vi "Echo.vi"(8 "error in (no error)":errorcluster, 10 "Error In":errorcluster, 11 "HandlerCore in":refnum<class "HandlerCore.lvclass">) -> (0 "error out":errorcluster, 1 "Still Pass?":bool, 2 "handled?":bool, 3 "HandlerCore out":refnum<class "HandlerCore.lvclass">)   [LabVIEW 2014, in "Chain Of Responsibility Pattern.lvlib" / "HandlerCore.lvclass"]
uses:
  HandlerCore.lvclass
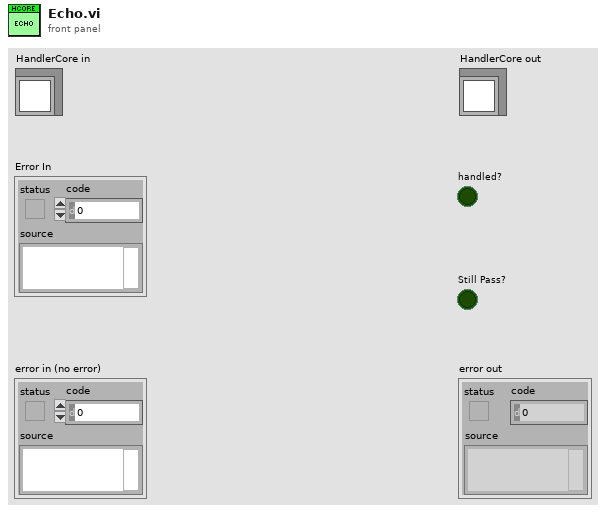
[diagram p1: front panel]
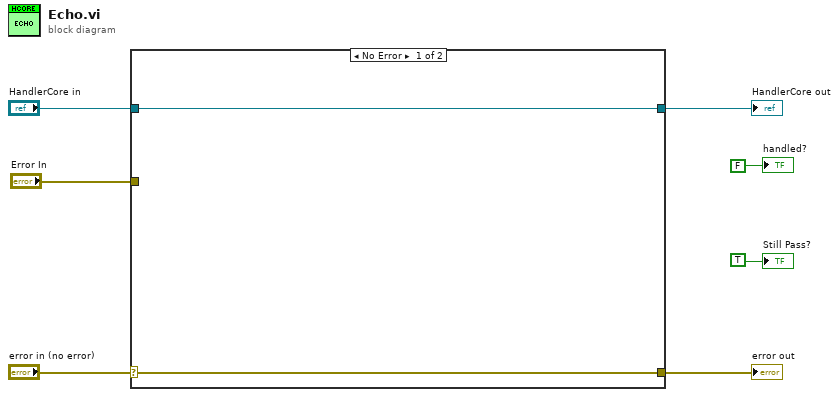
[diagram p0: block diagram]
diagram:
  n1 = case shown="No Error" "error in (no error)" {
    selector: "error in (no error)" -> [w8 w11]
    tunnel: [w8 w11] -> w6
    tunnel: [w9 w10] -> w4
    tunnel: "HandlerCore in" -> [w9 w10]
    tunnel: "Error In" -> [_ _]
    frame No Error {
    }
    frame Error {
    }
  }
  "error out" <- w6
  "HandlerCore out" <- w4
  "Still Pass?" <- TRUE
  "handled?" <- FALSE
